vi "PPScanPositionDefinition.vi"() -> (3 "Array":dbl[][](array[numeric]))   [LabVIEW 2017]
doc: "Use this template to build a user interface event handler design pattern. Use this pattern for dialog boxes and other user interfaces. You also can create and execute user-defined events that the VI can handle the same way as user interface events."
panel:
  in  "OK Button":bool
  in  "Pts in Y":dbl
  in  "Pts in X":dbl
  in  "dY (mm)":dbl
  in  "dX (mm)":dbl
  in  "Start Y (mm)":dbl
  in  "Start X (mm)":dbl
  # "Initial positions"
  # "Delta"
  # "Nbr of points"
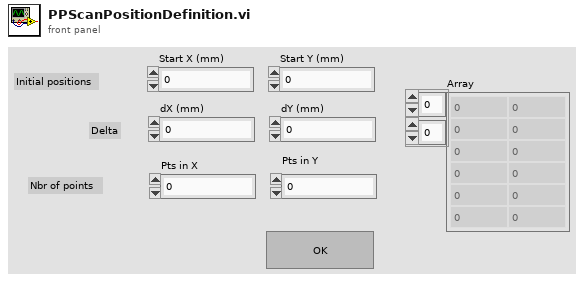
[diagram p1: front panel]
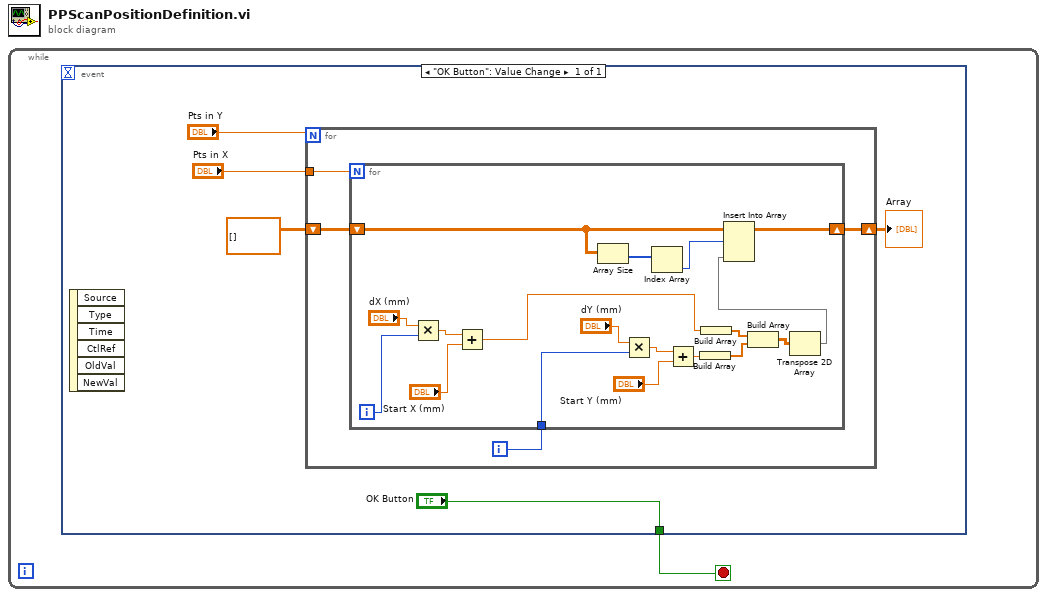
[diagram p0: block diagram]
diagram:
  n1 = while {
    stop <- w1 stop-if-true
    n2 = event shown="[0] \"OK Button\": Value Change" {
      selector: _ -> [_]
      dyn-events: _ -> [_]
      timeout: _ -> [_]
      tunnel: ["OK Button"] -> w1
      event "OK Button": Value Change {
        n3 = event-data() -> ()  [unwired: 1 in, 6 out]
        n4 = for {
          N: "Pts in Y" -> [_]
          tunnel: "Pts in X" -> [w10]
          shift-right: [w8] -> w2
          shift-left: dbl[][] [] -> [w7]
          i -> [w9]
          n5 = for {
            N: w10 -> [_]
            tunnel: w9 -> [w21]
            shift-right: [w16] -> w8
            shift-left: w7 -> [w13]
            i -> [w27]
            n6 = Multiply(x="dX (mm)", y=w27) -> (x*y=w25:dbl)
            n7 = Add(x=w25, y="Start X (mm)") -> (x+y=w17:dbl)
            n8 = Array Size(array=w13) -> (size(s)=w12:i32[])
            n9 = Multiply(x="dY (mm)", y=w21) -> (x*y=w24:dbl)
            n10 = Index Array(array=w12) -> (element=w11:i32)  [unwired: 1 in]
            n11 = Add(x=w24, y="Start Y (mm)") -> (x+y=w18:dbl)
            n12 = Build Array(w18) -> (w19:dbl[])
            n13 = Build Array(w17) -> (w20:dbl[])
            n14 = Build Array(w20, w19) -> (w15:dbl[][])
            n15 = Transpose 2D Array(2D array=w15) -> (transposed array=w14:dbl[][])
            n16 = Insert Into Array(array=w13, index (row)=w11, new element=w14) -> (w16:dbl[][])  [unwired: 1 in]
          }
        }
        "Array" <- w2
      }
    }
  }
